vi "Monta_Mensagem.vi"(1 "Zerar":bool, 2 "Mensagem":string) -> ()   [LabVIEW 2018]
uses:
  Global_Telescopio.vi
panel:
  in  "Numeric":i32
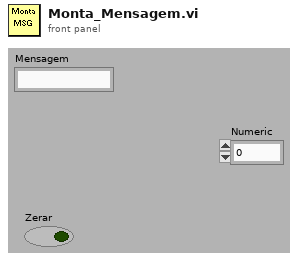
[diagram p1: front panel]
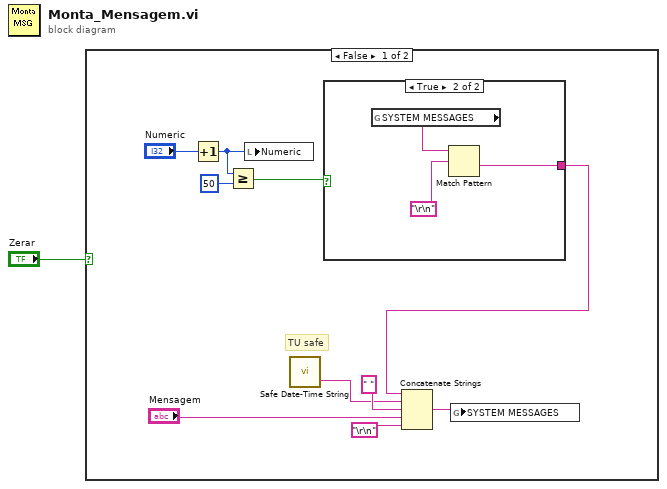
[diagram p0: block diagram]
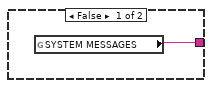
[diagram p2: hidden frame]
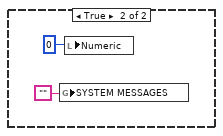
[diagram p3: hidden frame]
diagram:
  n1 = case shown="False" "Zerar" {
    frame False {
      # "TU safe"
      n2 = Increment(x="Numeric") -> (x+1=w6:i32)
      n3 = Greater Or Equal?(x=w6, y=50) -> (x >= y?=w4:bool)
      n4 = local write "Numeric"(w6) -> ()
      n5 = call "Safe Date-Time String.vi"() -> ("Safe time string"=w2:string)  [unwired: 3 in, 1 out]
      n6 = case shown="True" w4 {
        tunnel: [w12 w13] -> w3
        frame False {
          n7 = global read "Global_Telescopio.vi" "SYSTEM MESSAGES"() -> (w12:string)
        }
        frame True {
          n8 = global read "Global_Telescopio.vi" "SYSTEM MESSAGES"() -> (w14:string)
          n9 = Match Pattern(string=w14, regular expression="\r\n") -> (after substring=w13:string)  [unwired: 1 in, 3 out]
        }
      }
      n10 = Concatenate Strings(w3, w2, " " ("string"), "Mensagem", "\r\n") -> (w8:string)
      n11 = global write "Global_Telescopio.vi" "SYSTEM MESSAGES"(w8) -> ()
    }
    frame True {
      n12 = global write "Global_Telescopio.vi" "SYSTEM MESSAGES"("") -> ()
      n13 = local write "Numeric"(0 ("Numeric")) -> ()
    }
  }
